vi "Find and Replace SubVI.vi"(7 "Traverse Target":T1, 8 "error in (no error)":errorcluster, 9 "Old VI Name":string, 10 "New VI Path":path, 11 "vi reference in":refnum<vi>) -> (0 "error out":errorcluster, 2 "Replace":refnum<vi>, 3 "vi reference out":refnum<vi>)   [LabVIEW 2020, in "Message Maker.lvlib"]
uses:
  Message Maker.lvlib
  <vilib>/Utility/traverseref.llb/TRef TravTarget.ctl
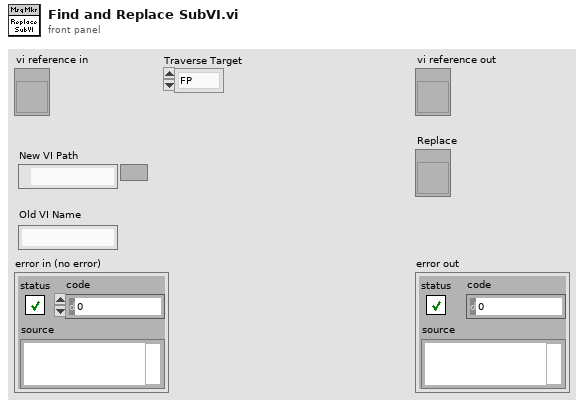
[diagram p1: front panel]
types:
  T1 = typedef "TRef TravTarget.ctl" = enum16{"FP", "BD", "Other"}
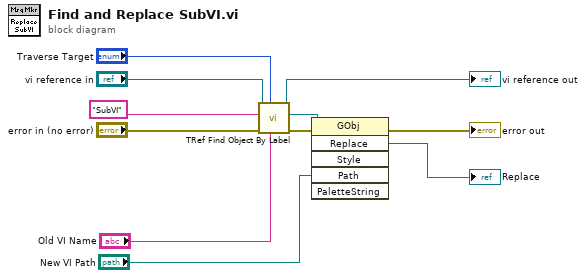
[diagram p0: block diagram]
diagram:
  n1 = call <vilib>:"TRef Find Object By Label.vi"("Label"="Old VI Name", "Traverse Target"="Traverse Target", "error in (no error)"="error in (no error)", "Class Name"="SubVI" ("GObj Class Name"), "VI Ref"="vi reference in") -> ("error out"=w1:errorcluster, "Found Obj Ref"=w2:refnum<vi>, "dup VI Ref"=→"vi reference out":refnum<vi>)  [unwired: 3 in, 1 out]
  n2 = invoke class="GObj" method="Replace"(reference=w2, error in=w1, "Path"="New VI Path") -> (error out=→"error out":errorcluster, "Replace"=→"Replace":refnum<vi>)  [unwired: 3 in, 4 out]
